vi "Logger Started.vi"(8 "error in (no error)":errorcluster, 10 "ID":string, 11 "Log Manager Module in":refnum<class "Log Manager Module.lvclass">) -> (0 "error out":errorcluster, 3 "Log Manager Module out":refnum<class "Log Manager Module.lvclass">)   [LabVIEW 2020, in "VolatusData.lvlib" / "Log Manager Module.lvclass"]
uses:
  Log Manager Module.lvclass
  Log Manager Module.lvclass/Log Manager Module.ctl
  Logger State.ctl
  VolatusData.lvlib
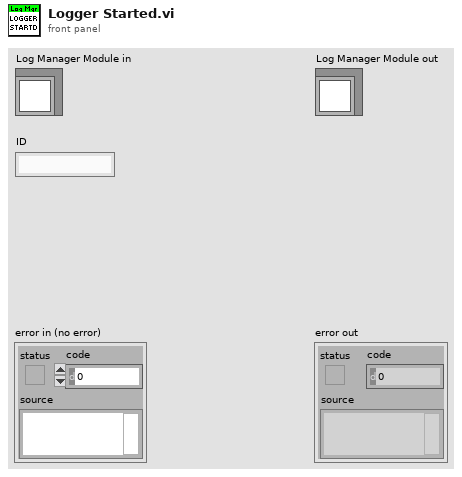
[diagram p1: front panel]
types:
  T1 = typedef "VolatusData.lvlib/Logger State.ctl" = enum16{"Unknown", "Idle", "Preparing", "Ready", "Logging", "Stopping"}
  T2 = typedef "VolatusData.lvlib/Log Manager Module.lvclass/Group Info.ctl" = cluster{"Name":string, "Loggers":map{string, T3}}
  T3 = typedef "VolatusData.lvlib/Log Manager Module.lvclass/Logger.ctl" = cluster{"ID":string, "MsgQ":refnum<class "MessageQ.lvclass">, "State":T1, "Group":string}
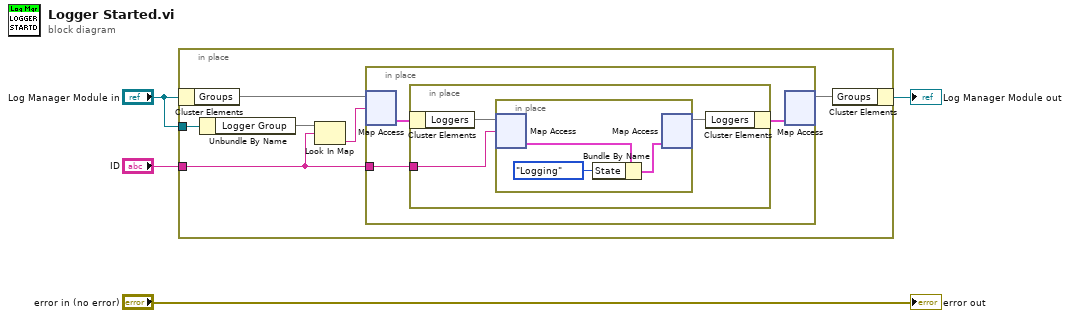
[diagram p0: block diagram]
diagram:
  n1 = in-place {
    in-place-border: "ID" -> [w8]
    in-place-border: "Log Manager Module in" -> [w10]
    n2 = in-place-cluster #1("Log Manager Module in") -> ("Groups"=w7:map{string, T2})
    n3 = Unbundle By Name(w10) -> ("Logger Group"=w9:map{string, string})
    n4 = Look In Map(map=w9, key=w8) -> (value=w6:string)  [unwired: 1 in, 1 out]
    n5 = in-place {
      in-place-border: w8 -> [w13]
      n6 = in-place-map #2(w7, w6) -> (w12:T2)  [unwired: 1 in, 1 out]
      n7 = in-place {
        in-place-border: w13 -> [w16]
        n8 = in-place-cluster #3(w12) -> ("Loggers"=w15:map{string, T3})
        n9 = in-place {
          n10 = in-place-map #4(w15, w16) -> (w19:T3)  [unwired: 1 in, 1 out]
          n11 = Bundle By Name(cluster=w19, "State"=Logger_State."Logging") -> (w17:T3)
          n12 = in-place-map #4(w17) -> (w14:map{string, T3})  [unwired: 1 in, 2 out]
        }
        n13 = in-place-cluster #3("Loggers"=w14) -> (w11:T2)
      }
      n14 = in-place-map #2(w11) -> (w5:map{string, T2})  [unwired: 1 in, 2 out]
    }
    n15 = in-place-cluster #1("Groups"=w5) -> (→"Log Manager Module out":refnum<class "Log Manager Module.lvclass">)
  }
  "error out" <- "error in (no error)"
